vi "FdxCmdTxUDPControlCvi.vi"(8 "error in":errorcluster, 9 "TxUdpControl":T1 {"NetSelect" items=["FDX_TX_FRAME_DLY_A"=0, "FDX_TX_FRAME_DLY_B"=1, "FDX_TX_FRAME_BOTH "=3, "FDX_TX_FRAME_ONLY_A"=4, "FDX_TX_FRAME_ONLY_B "=5]; "EnableTyp" items=["FDX_DIS", "FDX_ENA"]}, 11 "InstrumentHandle":u32) -> (0 "error out":errorcluster, 3 "InstrumentHandle":u32)   [LabVIEW 2020, in "AIM664LV.lvlib"]
doc: "This function is used to enable or disable a UDP Port and for error-injection purposes."
uses:
  AIM664LV.lvlib
  AFDX_LibraryAdmin/FdxGlobalDllPath.vi
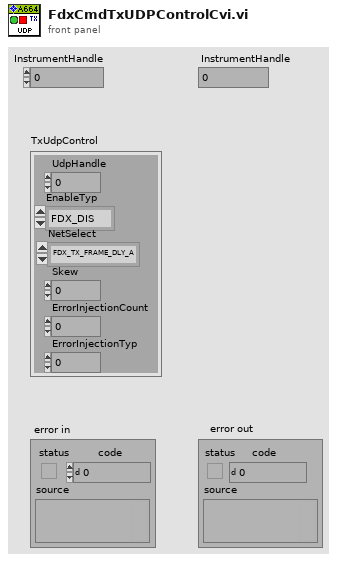
[diagram p1: front panel]
types:
  T1 = cluster{"UdpHandle":u32, "EnableTyp":u32, "NetSelect":u32, "Skew":u32, "ErrorInjectionCount":u32, "ErrorInjectionTyp":u32}
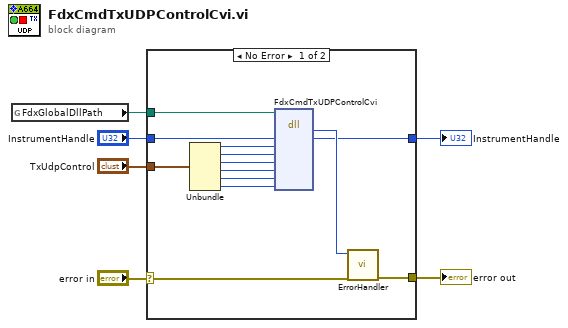
[diagram p0: block diagram]
diagram:
  n1 = global read "FdxGlobalDllPath.vi" "FdxGlobalDllPath"() -> (w4:path)
  n2 = case shown="No Error" "error in" {
    selector: "error in" -> [w18 w21]
    tunnel: [w19 w21] -> w6
    tunnel: w4 -> [w10 _]
    tunnel: "InstrumentHandle" -> [w9 w20]
    tunnel: [w8 w20] -> w2
    tunnel: "TxUdpControl" -> [w7 _]
    frame No Error {
      n3 = Unbundle(w7) -> ("UdpHandle"=w16:u32, "EnableTyp"=w15:u32, "NetSelect"=w14:u32, "Skew"=w13:u32, "ErrorInjectionCount"=w12:u32, "ErrorInjectionTyp"=w11:u32)
      n4 = dll-call lib="aim_fdx.19.dll" fn="FdxCmdTxUDPControlCvi"(path in=w10, "InstrumentHandle"=w9, "UdpHandle"=w16, "EnableTyp"=w15, "NetSelect"=w14, "Skew"=w13, "ErrorInjectionCount"=w12, "ErrorInjectionTyp"=w11) -> ("status"=w17:i32, "InstrumentHandle"=w8:u32)  [unwired: 8 in, 2 out]
      n5 = call "ErrorHandler.vi"("error in"=w18, "AIM Error"=w17) -> ("error out"=w19:errorcluster)  [unwired: 9 in]
    }
    frame Error {
    }
  }
  "error out" <- w6
  "InstrumentHandle" <- w2
